vi "CVT I32 GetIndex.vi"(8 "error in (no error)":errorcluster, 11 "Tag Name":string) -> (0 "error out":errorcluster, 3 "Tag Index":i32)   [LabVIEW 2016]
uses:
  <vilib>/NI/Current Value Table/DataTypes/I32_Get Index.vi
  <vilib>/NI/Current Value Table/Type to Enum.vi
  <vilib>/NI/Current Value Table/DataTypes/I32_Type To Enum.vi
  <vilib>/NI/Current Value Table/FGVs/Tag Memory.vi
  <vilib>/NI/Current Value Table/Current Value Table.lvlib
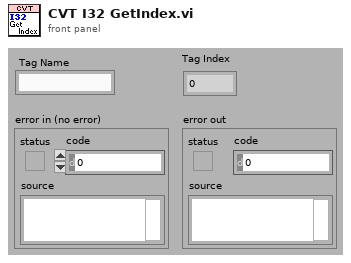
[diagram p1: front panel]
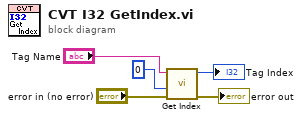
[diagram p0: block diagram]
diagram:
  n1 = call-poly <vilib>:"Get Index.vi"("error in (no error)"="error in (no error)", "Default"=0 ("Data Type"), "Tag Name"="Tag Name") -> ("error out"=→"error out":errorcluster, "Index"=→"Tag Index":i32)  [unwired: 7 in]
